vi "flipYZsgl.vi"(10 "pointIn":cluster{"X":sgl, "Y":sgl, "Z":sgl}) -> (2 "pointOut":cluster{"X":sgl, "Y":sgl, "Z":sgl})   [LabVIEW 2015]
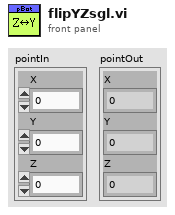
[diagram p1: front panel]
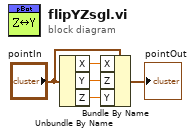
[diagram p0: block diagram]
diagram:
  n1 = Unbundle By Name("pointIn") -> ("X"=w4:sgl, "Y"=w3:sgl, "Z"=w2:sgl)
  n2 = Bundle By Name(cluster="pointIn", "X"=w4, "Z"=w3, "Y"=w2) -> (→"pointOut":cluster{"X":sgl, "Y":sgl, "Z":sgl})
